vi "Cleanup.vi"(8 "error in (no error)":errorcluster, 11 "Channel Buffer DBL in":refnum<class "Channel Buffer DBL.lvclass">) -> (0 "error out":errorcluster)   [LabVIEW 2020, in "VolatusHistorian.lvlib" / "Channel Buffer DBL.lvclass"]
uses:
  Channel Buffer DBL.lvclass
  Channel Buffer DBL.lvclass/Channel Buffer DBL.ctl
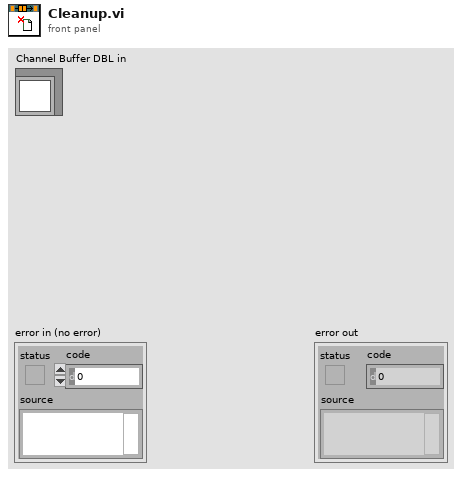
[diagram p1: front panel]
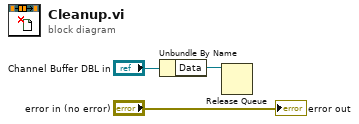
[diagram p0: block diagram]
diagram:
  n1 = Unbundle By Name("Channel Buffer DBL in") -> ("Data"=w1:refnum<queue>)
  n2 = Release Queue(queue=w1) -> ()  [unwired: 2 in, 3 out]
  "error out" <- "error in (no error)"
